vi "copy.vi"(8 "error in (no error)":errorcluster, 10 "ScriptEventForCopy":refnum<class "ScriptEvent.lvclass">, 11 "RampEvent in":refnum<class "RampEvent.lvclass">) -> (0 "error out":errorcluster, 3 "RampEvent Copy":refnum<class "RampEvent.lvclass">)   [LabVIEW 2011, in "Tools.lvlib" / "Scripting.lvlib" / "RampEvent.lvclass"]
uses:
  RampEvent.lvclass
  ScriptEvent.lvclass
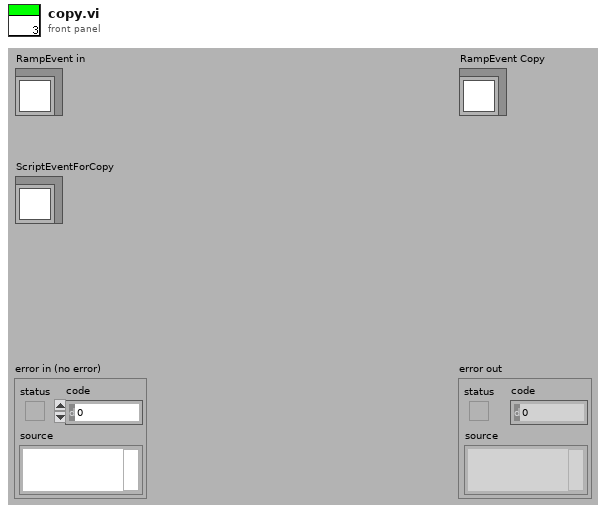
[diagram p1: front panel]
types:
  T1 = enum16{"changeValue", "pulse", "clock", "rampUp", "rampDown", "singleTone", "singleToneRamp", "playFile", "rf", "rfRamp", "delay"}
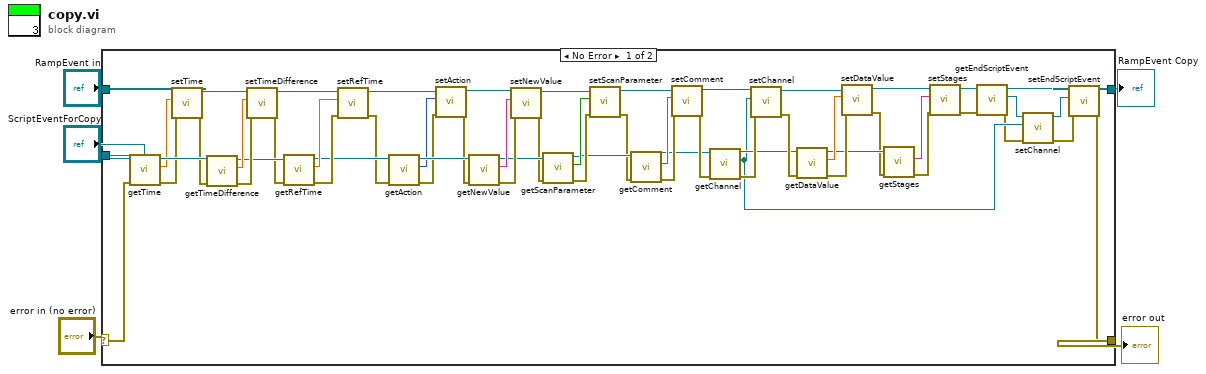
[diagram p0: block diagram]
diagram:
  n1 = case shown="No Error" "error in (no error)" {
    selector: "error in (no error)" -> [w24 w65]
    tunnel: "RampEvent in" -> [w33 w66]
    tunnel: [w16 w66] -> w2
    tunnel: [w14 w65] -> w1
    tunnel: "ScriptEventForCopy" -> [w64 _]
    frame No Error {
      n2 = call "getTime.vi"("error in (no error)"=w24, "ScriptEvent.lvclass in"=w64) -> ("error out"=w62:errorcluster, "time"=w61:dbl, "ScriptEvent.lvclass out"=w63:refnum<class "ScriptEvent.lvclass">)  [unwired: 7 in]
      n3 = call "setTime.vi"("error in (no error)"=w62, "time"=w61, "ScriptEvent.lvclass in"=w33) -> ("error out"=w60:errorcluster, "ScriptEvent.lvclass out"=w31:refnum<class "RampEvent.lvclass">)  [unwired: 7 in]
      n4 = call "getTimeDifference.vi"("error in (no error)"=w60, "ScriptEvent.lvclass in"=w63) -> ("error out"=w59:errorcluster, "time difference"=w32:dbl, "ScriptEvent.lvclass out"=w11:refnum<class "ScriptEvent.lvclass">)  [unwired: 7 in]
      n5 = call "setTimeDifference.vi"("error in (no error)"=w59, "time difference"=w32, "ScriptEvent.lvclass in"=w31) -> ("error out"=w10:errorcluster, "ScriptEvent.lvclass out"=w12:refnum<class "RampEvent.lvclass">)  [unwired: 7 in]
      n6 = call "getRefTime.vi"("error in (no error)"=w10, "ScriptEvent.lvclass in"=w11) -> ("error out"=w8:errorcluster, "refTime"=w9:dbl, "ScriptEvent.lvclass out"=w7:refnum<class "ScriptEvent.lvclass">)  [unwired: 7 in]
      n7 = call "setRefTime.vi"("error in (no error)"=w8, "refTime"=w9, "ScriptEvent.lvclass in"=w12) -> ("error out"=w6:errorcluster, "ScriptEvent.lvclass out"=w13:refnum<class "RampEvent.lvclass">)  [unwired: 7 in]
      n8 = call "getAction.vi"("error in (no error)"=w6, "ScriptEvent.lvclass in"=w7) -> ("error out"=w57:errorcluster, "action"=w56:T1, "ScriptEvent.lvclass out"=w58:refnum<class "ScriptEvent.lvclass">)  [unwired: 7 in]
      n9 = call "setAction.vi"("error in (no error)"=w57, "action"=w56, "ScriptEvent.lvclass in"=w13) -> ("error out"=w55:errorcluster, "ScriptEvent.lvclass out"=w30:refnum<class "RampEvent.lvclass">)  [unwired: 7 in]
      n10 = call "getNewValue.vi"("error in (no error)"=w55, "ScriptEvent.lvclass in"=w58) -> ("error out"=w54:errorcluster, "newValue"=w53:string, "ScriptEvent.lvclass out"=w52:refnum<class "ScriptEvent.lvclass">)  [unwired: 7 in]
      n11 = call "setNewValue.vi"("error in (no error)"=w54, "newValue"=w53, "ScriptEvent.lvclass in"=w30) -> ("error out"=w51:errorcluster, "ScriptEvent.lvclass out"=w29:refnum<class "RampEvent.lvclass">)  [unwired: 7 in]
      n12 = call "getScanParameter.vi"("error in (no error)"=w51, "ScriptEvent.lvclass in"=w52) -> ("error out"=w49:errorcluster, "scanParameter"=w50:bool, "ScriptEvent.lvclass out"=w48:refnum<class "ScriptEvent.lvclass">)  [unwired: 7 in]
      n13 = call "setScanParameter.vi"("error in (no error)"=w49, "scanParameter"=w50, "ScriptEvent.lvclass in"=w29) -> ("error out"=w47:errorcluster, "ScriptEvent.lvclass out"=w28:refnum<class "RampEvent.lvclass">)  [unwired: 7 in]
      n14 = call "getComment.vi"("error in (no error)"=w47, "ScriptEvent.lvclass in"=w48) -> ("error out"=w46:errorcluster, "comment"=w45:string, "ScriptEvent.lvclass out"=w43:refnum<class "ScriptEvent.lvclass">)  [unwired: 7 in]
      n15 = call-dynamic "setComment.vi"("error in (no error)"=w46, "comment"=w45, "RampEvent.lvclass in"=w28) -> ("error out"=w44:errorcluster, "RampEvent.lvclass out"=w27:refnum<class "RampEvent.lvclass">)  [unwired: 7 in]
      n16 = call-dynamic "getChannel.vi"("error in (no error)"=w44, "ScriptEvent.lvclass in"=w43) -> ("error out"=w42:errorcluster, "Channel.lvclass"=w19:refnum<class "Channel.lvclass">, "ScriptEvent.lvclass out"=w40:refnum<class "ScriptEvent.lvclass">)  [unwired: 7 in]
      n17 = call-dynamic "setChannel.vi"("error in (no error)"=w42, "Channel.lvclass"=w19, "RampEvent.lvclass in"=w27) -> ("error out"=w41:errorcluster, "RampEvent.lvclass out"=w26:refnum<class "RampEvent.lvclass">)  [unwired: 7 in]
      n18 = call "getDataValue.vi"("error in (no error)"=w41, "ScriptEvent.lvclass in"=w40) -> ("error out"=w39:errorcluster, "dataValue"=w38:dbl, "ScriptEvent.lvclass out"=w37:refnum<class "ScriptEvent.lvclass">)  [unwired: 7 in]
      n19 = call "setDataValue.vi"("error in (no error)"=w39, "dataValue"=w38, "ScriptEvent.lvclass in"=w26) -> ("error out"=w36:errorcluster, "ScriptEvent.lvclass out"=w25:refnum<class "RampEvent.lvclass">)  [unwired: 7 in]
      n20 = call "getStages.vi"("error in (no error)"=w36, "ScriptEvent.lvclass in"=w37) -> ("error out"=w35:errorcluster, "Stage"=w34:string)  [unwired: 7 in, 1 out]
      n21 = call-dynamic "setStages.vi"("error in (no error)"=w35, "Stage"=w34, "RampEvent.lvclass in"=w25) -> ("error out"=w22:errorcluster, "RampEvent.lvclass out"=w23:refnum<class "RampEvent.lvclass">)  [unwired: 7 in]
      n22 = call "getEndScriptEvent.vi"("error in (no error)"=w22, "RampEvent.lvclass in"=w23) -> ("error out"=w18:errorcluster, "ScriptEvent.lvclass"=w20:refnum<class "ScriptEvent.lvclass">, "RampEvent.lvclass out"=w21:refnum<class "RampEvent.lvclass">)  [unwired: 7 in]
      n23 = call-dynamic "setChannel.vi"("error in (no error)"=w18, "Channel.lvclass"=w19, "ScriptEvent.lvclass in"=w20) -> ("error out"=w15:errorcluster, "ScriptEvent.lvclass out"=w17:refnum<class "ScriptEvent.lvclass">)  [unwired: 7 in]
      n24 = call "setEndScriptEvent.vi"("error in (no error)"=w15, "endScriptEvent.lvclass"=w17, "RampEvent.lvclass in"=w21) -> ("error out"=w14:errorcluster, "RampEvent.lvclass out"=w16:refnum<class "RampEvent.lvclass">)  [unwired: 7 in]
    }
    frame Error {
    }
  }
  "error out" <- w1
  "RampEvent Copy" <- w2
